vi "Cycle.vi"(8 "error in (no error)":errorcluster, 11 "WhiteNoiseOrientationDetection In":refnum<class "WhiteNoiseOrientationDetection.lvclass">) -> (0 "error out":errorcluster, 3 "WhiteNoiseOrientationDetection Out":refnum<class "WhiteNoiseOrientationDetection.lvclass">)   [LabVIEW 2012, in "WhiteNoiseOrientationDetection.lvclass"]
uses:
  WhiteNoiseOrientationDetection.lvclass
  WhiteNoiseOrientationDetection.lvclass/WhiteNoiseOrientationDetection.ctl
  Trial Based Experiment Statechart/MatlabExperiment/MatlabExperiment.lvclass
panel:
  out "InResponseWindow":bool
  in  "targetFixationRadius":dbl=50.0
  in  "nFramesCoh":dbl=500.0
  in  "nFramesPreMax":dbl=500.0
  in  "nFramesPreMean":dbl=200.0
  in  "nFramesPreMin":dbl=50.0
  in  "responseInterval":dbl=2000.0 max=10000.0
  in  "Eye Params":dbl[](array[numeric])
  out "XY Graph":cluster{dbl[], dbl[]}(graph)
  in  "RewardAmount":dbl=50.0
  in  "FixationRadius":dbl=50.0
  out "Timeouts":T1={"Intertrial"=1000.0, "AcquireFixation"=1000.0, "HoldFixation"=300.0, "DelayPeriod"=1000.0, "ResponsePeriod"=1000.0}
  out "ExperimentStats":T2
  out "Cycles":dbl
  # "This is only used on labview and stored\non matlab.  The time window in which he can\nmake a correct response."
  # "Fuck"
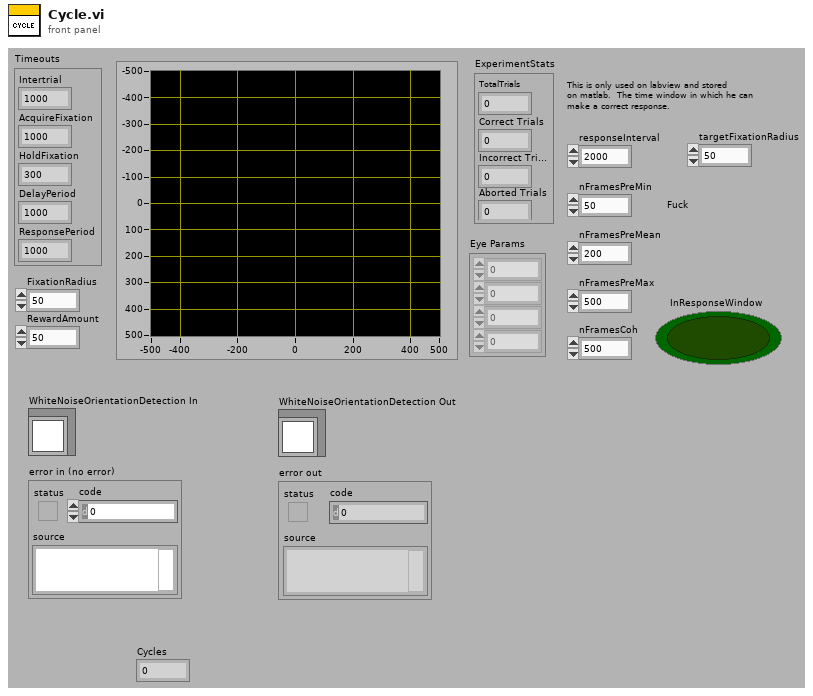
[diagram p1: front panel]
types:
  T1 = cluster{"Intertrial":dbl, "AcquireFixation":dbl, "HoldFixation":dbl, "DelayPeriod":dbl, "ResponsePeriod":dbl}
  T2 = cluster{"TotalTrials":dbl, "Correct Trials":dbl, "Incorrect Trials":dbl, "Aborted Trials":dbl}
  T3 = cluster{"TotalTrials":u32, "Correct Trials":u32, "Incorrect Trials":u32, "Aborted Trials":u32}
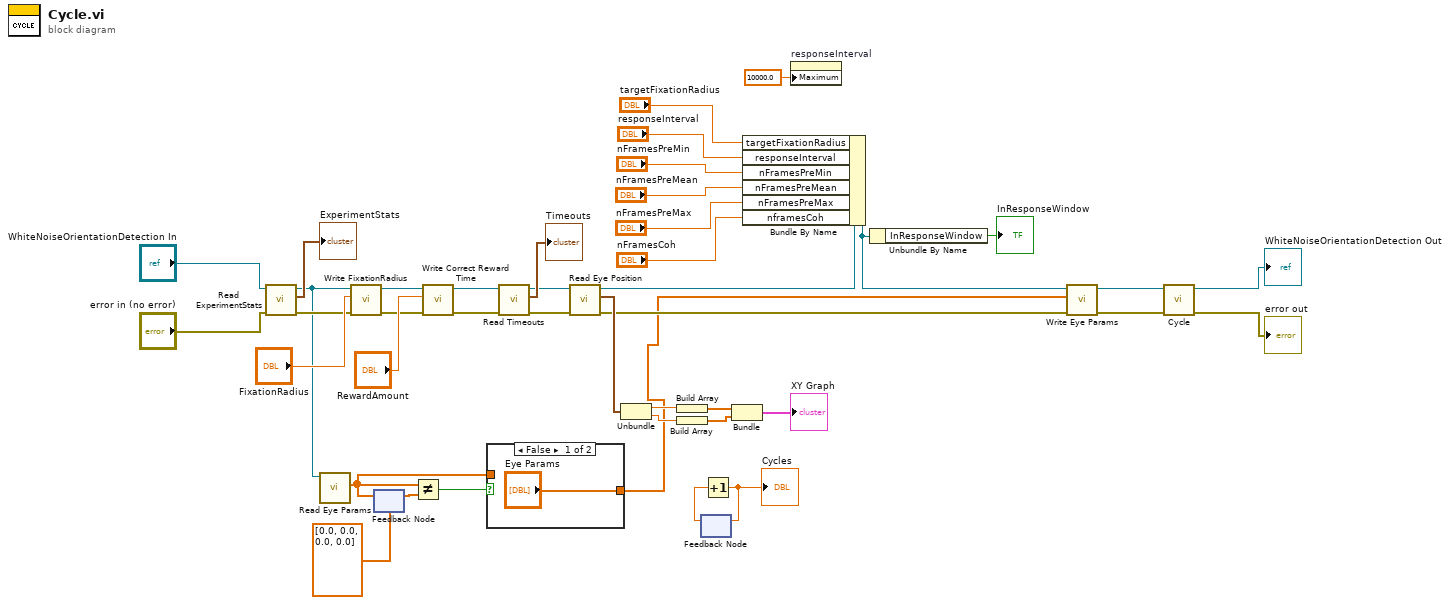
[diagram p0: block diagram]
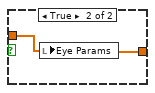
[diagram p2: hidden frame]
diagram:
  n1 = call-dynamic "Read ExperimentStats.vi"("error in (no error)"="error in (no error)", "TrialBasedExperiment in"="WhiteNoiseOrientationDetection In") -> ("error out"=w34:errorcluster, "ExperimentStats"=→"ExperimentStats":T3, "TrialBasedExperiment out"=w20:refnum<class "WhiteNoiseOrientationDetection.lvclass">)  [unwired: 7 in]
  n2 = call-dynamic "Read Eye Params.vi"("TrialBasedExperiment in"=w20) -> ("Eye Params"=w17:dbl[])  [unwired: 8 in, 2 out]
  n3 = call-dynamic "Write FixationRadius.vi"("error in (no error)"=w34, "FixationRadius"="FixationRadius", "MatlabExperiment in"=w20) -> ("error out"=w33:errorcluster, "MatlabExperiment out"=w36:refnum<class "WhiteNoiseOrientationDetection.lvclass">)  [unwired: 7 in]
  n4 = feedback #1(dbl[] [0.0, 0.0, 0.0, 0.0] ("Eye Params")) -> (w19:dbl[])
  n5 = feedback-in #1(w17) -> ()
  n6 = Not Equal?(x=w17, y=w19) -> (x != y?=w18:bool)
  n7 = call-dynamic "Write Correct Reward Time.vi"("error in (no error)"=w33, "Correct Reward Time"="RewardAmount", "MatlabExperiment in"=w36) -> ("error out"=w32:errorcluster, "MatlabExperiment out"=w35:refnum<class "WhiteNoiseOrientationDetection.lvclass">)  [unwired: 7 in]
  n8 = case shown="False" w18 {
    tunnel: w17 -> [_ w44]
    tunnel: ["Eye Params" w44] -> w16
    frame False {
    }
    frame True {
      n9 = local write "Eye Params"(w44) -> ()
    }
  }
  n10 = call-dynamic "Read Timeouts.vi"("error in (no error)"=w32, "TrialBasedExperiment in"=w35) -> ("error out"=w24:errorcluster, "Timeouts"=→"Timeouts":T1, "TrialBasedExperiment out"=w25:refnum<class "WhiteNoiseOrientationDetection.lvclass">)  [unwired: 7 in]
  n11 = call-dynamic "Read Eye Position.vi"("error in (no error)"=w24, "TrialBasedExperiment in"=w25) -> ("error out"=w23:errorcluster, "Eye Position"=w31:cluster{"Horizontal":dbl, "Vertical":dbl}, "TrialBasedExperiment out"=w10:refnum<class "WhiteNoiseOrientationDetection.lvclass">)  [unwired: 7 in]
  n12 = Unbundle(w31) -> ("Horizontal"=w30:dbl, "Vertical"=w29:dbl)
  n13 = Build Array(w30) -> (w28:dbl[])
  n14 = Build Array(w29) -> (w27:dbl[])
  n15 = feedback #2() -> (w41:dbl)  [unwired: 1 in]
  n16 = Increment(x=w41) -> (x+1=w42:dbl)
  "Cycles" <- w42
  n17 = feedback-in #2(w42) -> ()
  n18 = Bundle(w28, w27) -> (→"XY Graph":cluster{dbl[], dbl[]})  [unwired: 1 in]
  n19 = Bundle By Name(cluster=w10, "targetFixationRadius"="targetFixationRadius", "responseInterval"="responseInterval", "nFramesPreMin"="nFramesPreMin", "nFramesPreMean"="nFramesPreMean", "nFramesPreMax"="nFramesPreMax", "nframesCoh"="nFramesCoh") -> (w2:refnum<class "WhiteNoiseOrientationDetection.lvclass">)
  n20 = property on="responseInterval" class="DigNum (strict)"("Maximum"=10000.0 ("Data Entry Limits:Maximum")) -> ()  [unwired: 2 in, 2 out]
  n21 = Unbundle By Name(w2) -> ("InResponseWindow"=→"InResponseWindow":bool)
  n22 = call-dynamic "Write Eye Params.vi"("error in (no error)"=w23, "Eye Params"=w16, "TrialBasedExperiment in"=w2) -> ("error out"=w21:errorcluster, "TrialBasedExperiment out"=w22:refnum<class "WhiteNoiseOrientationDetection.lvclass">)  [unwired: 7 in]
  n23 = call-parent "Cycle.vi"("error in (no error)"=w21, "MatlabExperiment In"=w22) -> ("error out"=→"error out":errorcluster, "MatlabExperiment Out"=→"WhiteNoiseOrientationDetection Out":refnum<class "WhiteNoiseOrientationDetection.lvclass">)  [unwired: 8 in]
